vi "TCP-Write.vi"(8 "error in":errorcluster, 9 "data in":string, 10 "timeout ms (25000)":i32, 11 "Module ID":i32=-1) -> (0 "error out":errorcluster)   [LabVIEW 2018, in "TCP-IP Engine.lvlib"]
doc: "This Request event will request the TCP-IP Module to write the Data which is connected to the Data In terminal of the Input.\n_____\nCreated using DQMH Event Scripter 7.0.1.1316."
uses:
  TCP-IP Engine.lvlib
  TCP-Write Argument--cluster.ctl
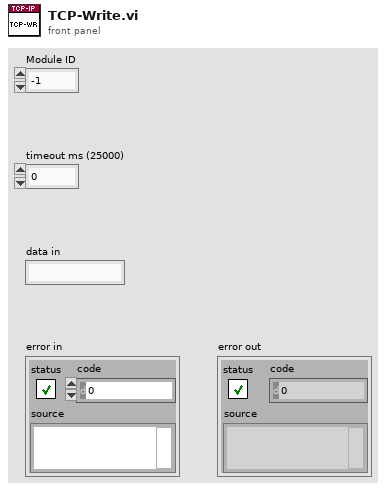
[diagram p1: front panel]
types:
  T1 = typedef "TCP-IP Engine.lvlib/TCP-Write Argument--cluster.ctl" = cluster{"Module ID":i32, "timeout ms (25000)":i32, "data in":string}
  T2 = typedef "TCP-IP Engine.lvlib/Request Events--cluster.ctl" = cluster{"Stop Module":refnum<user-event>, "Show Panel":refnum<user-event>, "Hide Panel":refnum<user-event>, "Show Diagram":refnum<user-event>, "Get Module Execution Status":refnum<user-event>, "TCP-Open Connection":refnum<user-event>, "Read TCP Data":refnum<user-event>, "TCP-Write":refnum<user-event>, "TCP-Close Connection":refnum<user-event>}
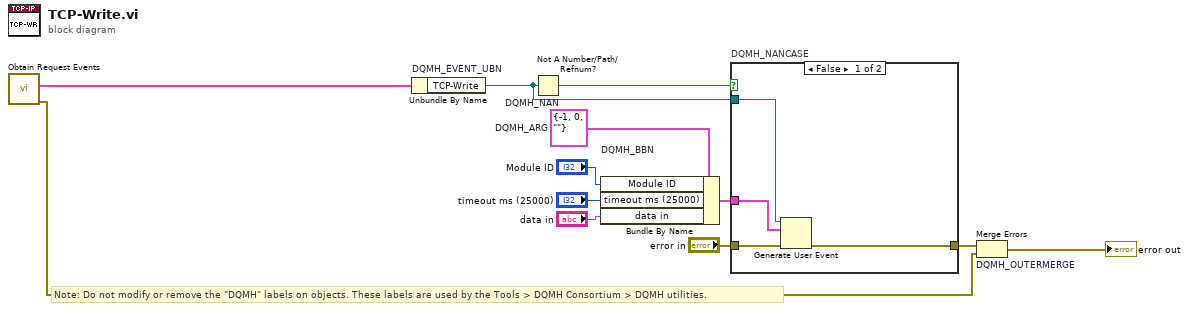
[diagram p0: block diagram]
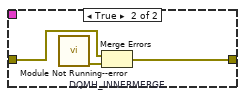
[diagram p2: hidden frame]
diagram:
  w6 = T1 {"Module ID"=-1, "timeout ms (25000)"=0, "data in"=""}  # DQMH_ARG
  # "Note: Do not modify or remove the \"DQMH\" labels on objects. These labels are used by the Tools > DQMH Consortium > DQMH utilities."
  n1 = call "Obtain Request Events.vi"() -> ("error out"=w2:errorcluster, "TCP-IP Engine Request Events"=w1:T2)  [unwired: 10 in]
  n2 = Unbundle By Name "DQMH_EVENT_UBN"(w1) -> ("TCP-Write"=w8:refnum<user-event>)
  n3 = Not A Number/Path/Refnum? "DQMH_NAN"(number/path/refnum=w8) -> (NaN/Path/Refnum?=w9:bool)
  n4 = Bundle By Name "DQMH_BBN"(cluster=w6, "Module ID"="Module ID", "timeout ms (25000)"="timeout ms (25000)", "data in"="data in") -> (w10:T1)
  n5 = case "DQMH_NANCASE" shown="False" w9 {
    tunnel: "error in" -> [w16 w19]
    tunnel: [w15 w18] -> w7
    tunnel: w8 -> [w14 _]
    tunnel: w10 -> [w13 _]
    frame False {
      n6 = Generate User Event(user event=w14, event data cluster=w13, error in=w16) -> (error out=w15:errorcluster)  [unwired: 1 in, 1 out]
    }
    frame True {
      n7 = call "Module Not Running--error.vi"() -> ("error out"=w17:errorcluster)  [unwired: 11 in]
      n8 = Merge Errors "DQMH_INNERMERGE"(w19, w17) -> (w18:errorcluster)
    }
  }
  n9 = Merge Errors "DQMH_OUTERMERGE"(w7, w2) -> (→"error out":errorcluster)
